vi "RepairLine.vi"(5 "Repair Line Col":bool, 7 "Repair Line Row":bool, 8 "Line Col":dbl, 9 "Line Row":dbl, 11 "Array In":dbl[][](array[numeric])) -> (3 "Array Repaired":dbl[][](array[numeric]))   [LabVIEW 2018]
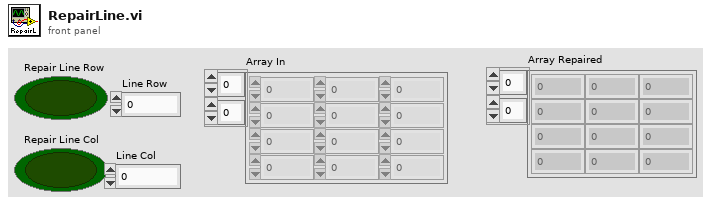
[diagram p1: front panel]
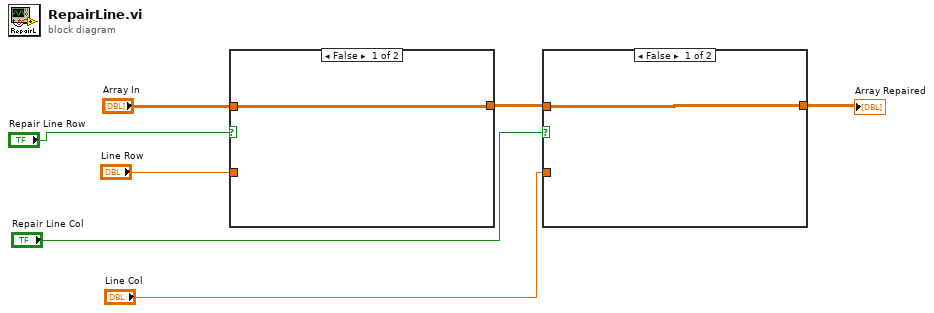
[diagram p0: block diagram]
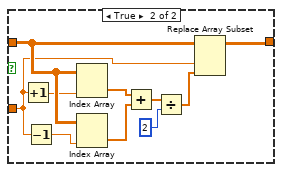
[diagram p2: hidden frame]
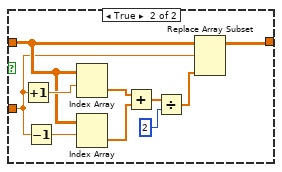
[diagram p3: hidden frame]
diagram:
  n1 = case shown="False" "Repair Line Row" {
    tunnel: "Line Row" -> [_ w9]
    tunnel: "Array In" -> [w8 w14]
    tunnel: [w8 w18] -> w5
    frame False {
    }
    frame True {
      n2 = Increment(x=w9) -> (x+1=w17:dbl)
      n3 = Decrement(x=w9) -> (x-1=w16:dbl)
      n4 = Index Array(array=w14, index (row)=w17) -> (element=w15:dbl[])  [unwired: 1 in]
      n5 = Index Array(array=w14, index (row)=w16) -> (element=w13:dbl[])  [unwired: 1 in]
      n6 = Add(x=w15, y=w13) -> (x+y=w12:dbl[])
      n7 = Divide(x=w12, y=2) -> (x/y=w10:dbl[])
      n8 = Replace Array Subset(array=w14, new element=w10, index (row)=w9) -> (w18:dbl[][])  [unwired: 1 in]
    }
  }
  n9 = case shown="False" "Repair Line Col" {
    tunnel: "Line Col" -> [_ w20]
    tunnel: w5 -> [w19 w27]
    tunnel: [w19 w29] -> w1
    frame False {
    }
    frame True {
      n10 = Increment(x=w20) -> (x+1=w22:dbl)
      n11 = Decrement(x=w20) -> (x-1=w21:dbl)
      n12 = Index Array(array=w27, index (col)=w22) -> (element=w28:dbl[])  [unwired: 1 in]
      n13 = Index Array(array=w27, index (col)=w21) -> (element=w26:dbl[])  [unwired: 1 in]
      n14 = Add(x=w28, y=w26) -> (x+y=w25:dbl[])
      n15 = Divide(x=w25, y=2) -> (x/y=w23:dbl[])
      n16 = Replace Array Subset(array=w27, new element=w23, index (col)=w20) -> (w29:dbl[][])  [unwired: 1 in]
    }
  }
  "Array Repaired" <- w1
